vi "PAN_GetAsyncN.vi"() -> (2 "asyncN":refnum<notifier>)   [LabVIEW 2016]
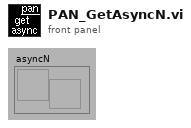
[diagram p1: front panel]
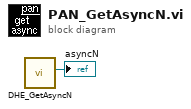
[diagram p0: block diagram]
diagram:
  n1 = call "DHE_GetAsyncN.vi"() -> ("asyncN"=→"asyncN":refnum<notifier>)  [unwired: 11 out]
